vi "makeDecisions.vi"(8 "error in (no error)":errorcluster, 10 "model":refnum<class "Model.lvclass">, 11 "EndingCycleState in":refnum<class "EndingCycleState.lvclass">) -> (0 "error out":errorcluster, 2 "model 2":refnum<class "Model.lvclass">, 3 "EndingCycleState out":refnum<class "EndingCycleState.lvclass">)   [LabVIEW 2013, in "EndingCycleState.lvclass"]
uses:
  EndingCycleState.lvclass
  Model/Model/Model.lvclass
  AutomatedProfileState/AutomatedProfileState.lvclass
  Typedefs/StateSelector.ctl
  Typedefs/FAMTTypedefs.lvlib
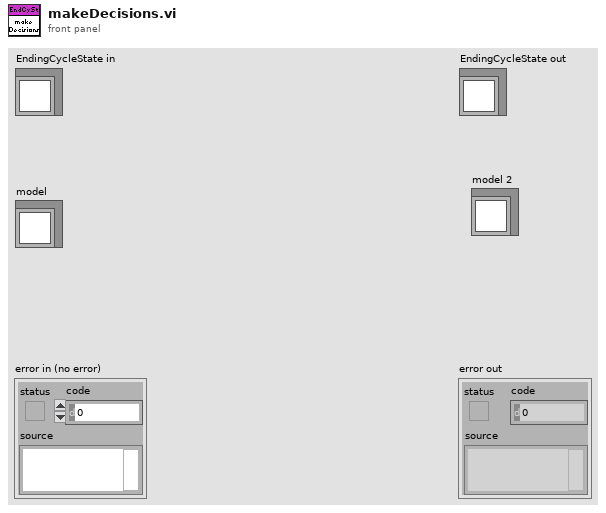
[diagram p1: front panel]
types:
  T1 = typedef "FAMTTypedefs.lvlib/StateSelector.ctl" = enum16{"EndingCycleState", "FaultState", "InteractiveSetpointState", "OffState", "StandbyState", "StoppedState"}
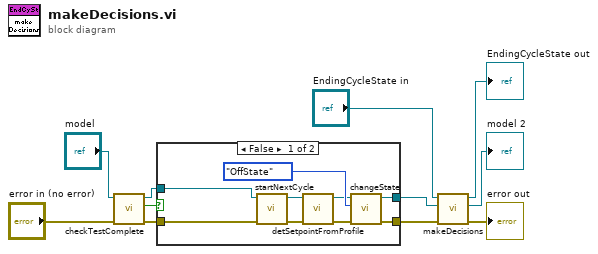
[diagram p0: block diagram]
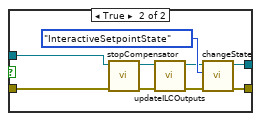
[diagram p2: hidden frame]
diagram:
  n1 = call "checkTestComplete.vi"("error in (no error)"="error in (no error)", "Model in"="model") -> ("error out"=w4:errorcluster, "testCompleteIsTrue"=w1:bool, "Model out"=w6:refnum<class "Model.lvclass">)  [unwired: 7 in]
  n2 = case shown="False" w1 {
    tunnel: w6 -> [w20 w29]
    tunnel: w4 -> [w18 w27]
    tunnel: [w17 w26] -> w3
    tunnel: [w19 w25] -> w2
    frame False {
      n3 = call "startNextCycle.vi"("error in (no error)"=w18, "Model in"=w20) -> ("error out"=w14:errorcluster, "Model out"=w15:refnum<class "Model.lvclass">)  [unwired: 8 in]
      n4 = call "detSetpointFromProfile.vi"("error in (no error)"=w14, "Model in"=w15) -> ("error out"=w12:errorcluster, "Model out"=w13:refnum<class "Model.lvclass">)  [unwired: 8 in]
      n5 = call "changeState.vi"("error in (no error)"=w12, "State:"=StateSelector."OffState", "Model in"=w13) -> ("error out"=w17:errorcluster, "Model out"=w19:refnum<class "Model.lvclass">)  [unwired: 7 in]
    }
    frame True {
      n6 = call "stopCompensator.vi"("error in (no error)"=w27, "Model in"=w29) -> ("error out"=w23:errorcluster, "Model out"=w24:refnum<class "Model.lvclass">)  [unwired: 8 in]
      n7 = call "updateILCOutputs.vi"("error in (no error)"=w23, "Model in"=w24) -> ("error out"=w21:errorcluster, "Model out"=w22:refnum<class "Model.lvclass">)  [unwired: 8 in]
      n8 = call "changeState.vi"("error in (no error)"=w21, "State:"=StateSelector."InteractiveSetpointState", "Model in"=w22) -> ("error out"=w26:errorcluster, "Model out"=w25:refnum<class "Model.lvclass">)  [unwired: 7 in]
    }
  }
  n9 = call-parent "makeDecisions.vi"("error in (no error)"=w3, "model"=w2, "EnabledState in"="EndingCycleState in") -> ("error out"=→"error out":errorcluster, "model 2"=→"model 2":refnum<class "Model.lvclass">, "EnabledState out"=→"EndingCycleState out":refnum<class "EndingCycleState.lvclass">)  [unwired: 6 in]
